vi "getSigProcessing.vi"(0 "Analogue Data (volts)":dbl[][](array[numeric])) -> (1 "Labelled Signals":string[][](array[string]), 2 "Channel Names":string[](array[string]), 3 "Raw Signals":dbl[][](array[numeric]))   [LabVIEW 2013]
uses:
  Globals/measurementGlobal.vi
panel:
  out "Chell Chans.":dbl[](array[numeric])
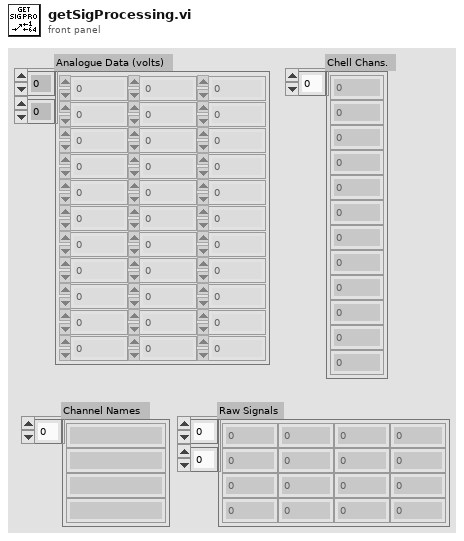
[diagram p1: front panel]
types:
  T1 = typedef "chanType.ctl" = enum16{"Default", "Clock", "Pressure Scanner"}
  T2 = typedef "chanData.ctl" = cluster{"Raw Data":dbl[], "Channel Name":string}
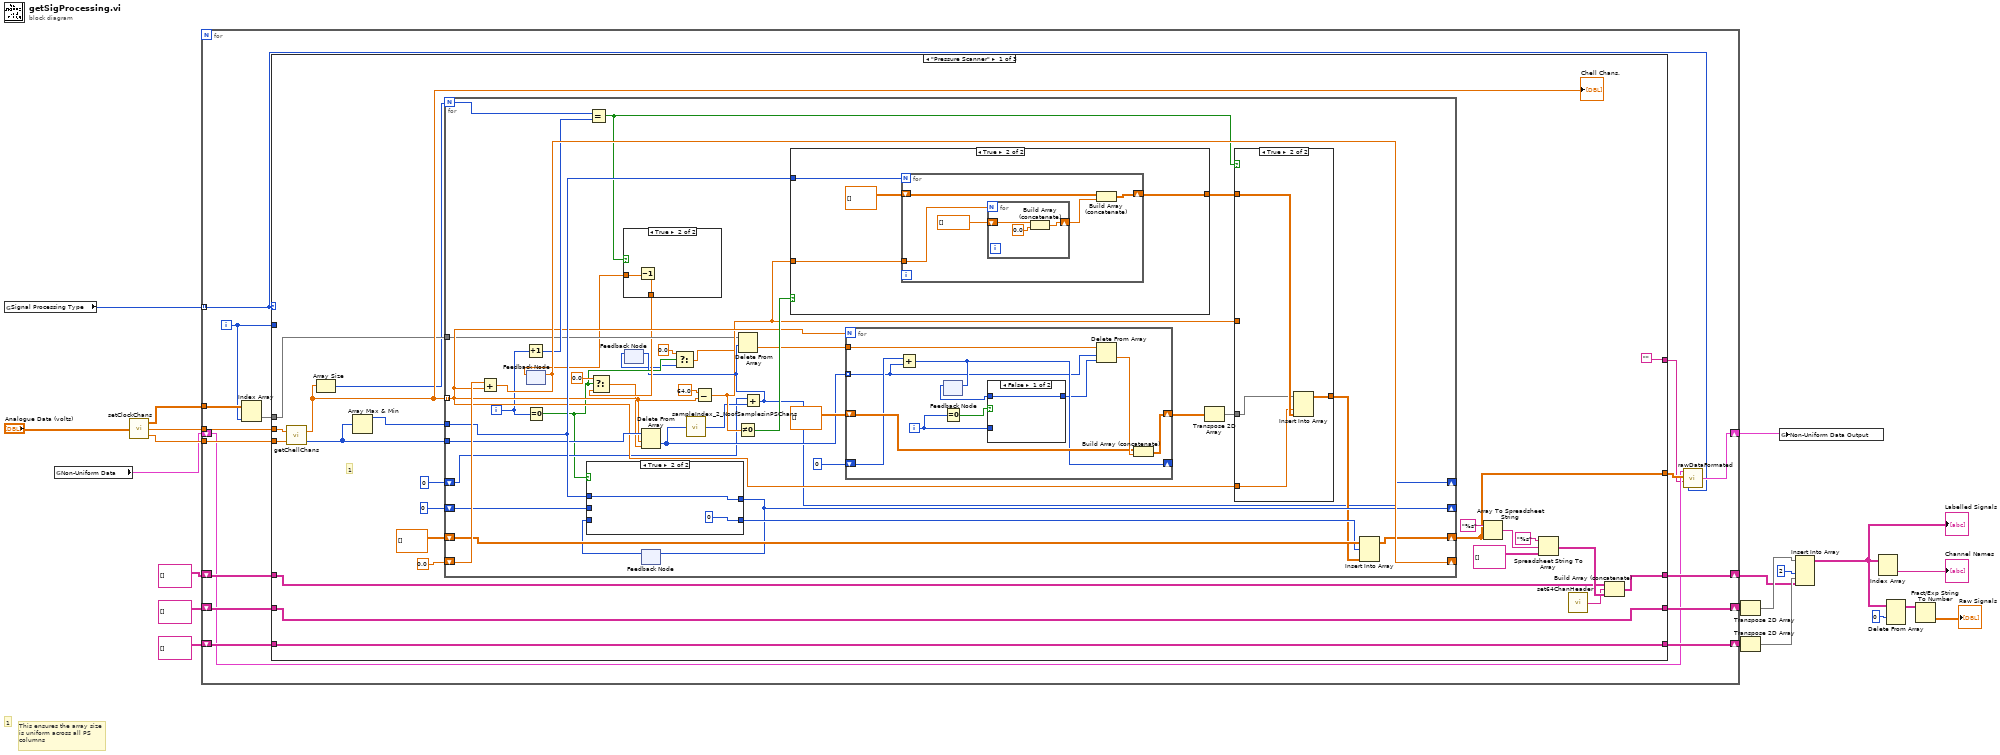
[diagram p0: block diagram]
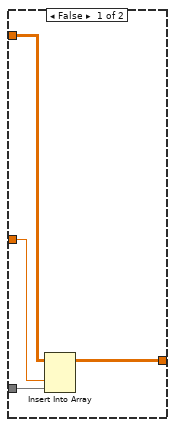
[diagram p3: hidden frame]
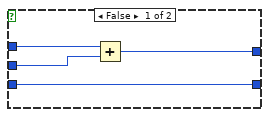
[diagram p4: hidden frame]
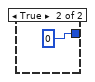
[diagram p5: hidden frame]
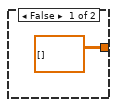
[diagram p6: hidden frame]
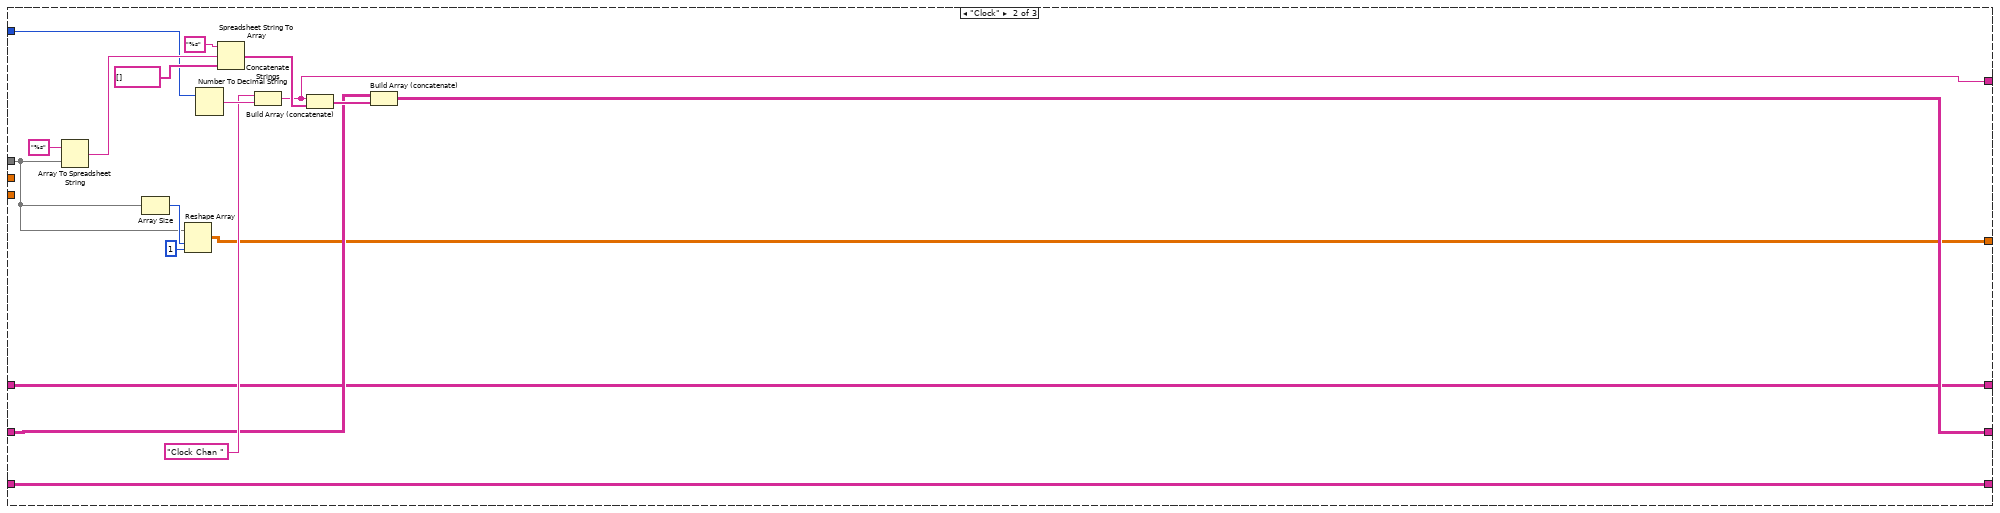
[diagram p7: hidden frame]
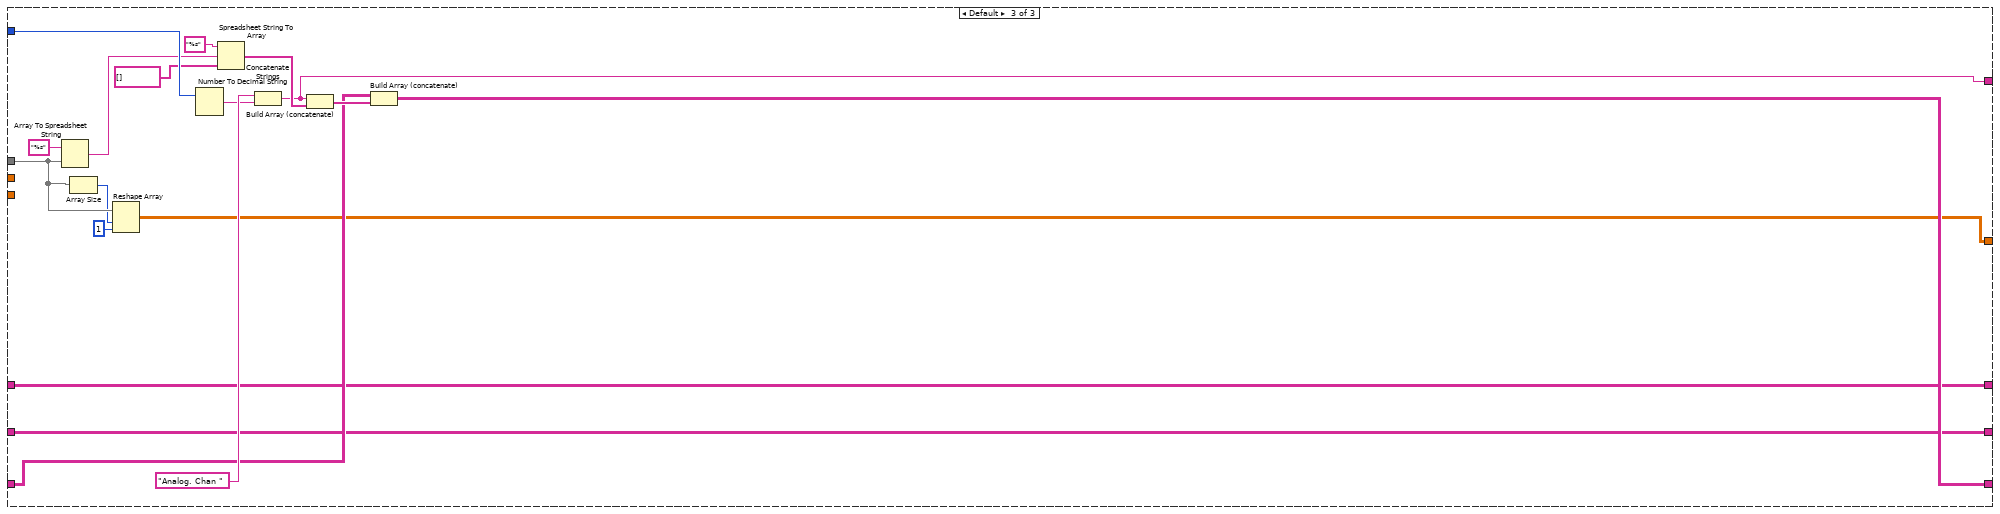
[diagram p8: hidden frame]
diagram:
  # "1"
  # "This ensures the array size\nis uniform across all PS\ncolumns"
  n1 = global read "measurementGlobal.vi" "Signal Processing Type"() -> (w21:T1[])
  n2 = global read "measurementGlobal.vi" "Non-Uniform Data"() -> (w2:T2[])
  n3 = call "setClockChans.vi"("Analogue Data (volts)"="Analogue Data (volts)") -> ("Modified Analogue Data (volts)"=w14:dbl[][], "MSB"=w13:dbl[], "LSB"=w12:dbl[])
  n4 = for {
    tunnel: w21 -> [w22] mode=indexing
    tunnel: w14 -> [w36]
    tunnel: w13 -> [w35]
    tunnel: w12 -> [w34]
    shift-right: [w31] -> w9
    shift-left: string[][] [] -> [w32]
    shift-right: [w29] -> w5
    shift-left: string[][] [] -> [w30]
    shift-right: [w27] -> w3
    shift-left: string[][] [] -> [w28]
    shift-right: [w25] -> w1
    shift-left: w2 -> [w24]
    i -> [w33]
    n5 = Index Array(array=w36, index (col)=w33) -> (element=w37:dbl[])  [unwired: 1 in]
    n6 = case shown="\"Pressure Scanner\"" w22 {
      tunnel: w37 -> [w52 w144 w163]
      tunnel: w35 -> [w60 _ _]
      tunnel: w34 -> [w59 _ _]
      tunnel: w33 -> [_ w152 w176]
      tunnel: w32 -> [w46 w150 w166]
      tunnel: [w46 w149 w166] -> w31
      tunnel: w30 -> [w45 w148 w168]
      tunnel: [w45 w148 w167] -> w29
      tunnel: w28 -> [w44 w147 w165]
      tunnel: [w43 w147 w165] -> w27
      tunnel: [w40 w143 w161] -> w26
      tunnel: ["" w142 w160] -> w23
      frame "Pressure Scanner" {
        # "1"
        n7 = call "getChellChans.vi"("LSB"=w59, "MSB"=w60) -> ("Sample Index"=w58:i32[], "No. Chell Chans."=w55:dbl[])
        "Chell Chans." <- w55
        n8 = Array Size(array=w55) -> (size(s)=w42:i32)
        n9 = Array Max & Min(array=w58) -> (max value=w57:i32)  [unwired: 3 out]
        n10 = for {
          N: w42 -> [w85]
          tunnel: w55 -> [w82] mode=indexing
          tunnel: w52 -> [w77]
          tunnel: w58 -> [w87]
          tunnel: w57 -> [w92]
          shift-right: [w94] -> _
          shift-left: 0.0 -> [w95]
          shift-right: [w61] -> w40
          shift-left: dbl[][] [] ("array") -> [w93]
          shift-right: [w89] -> _
          shift-left: 0 -> [w90]
          shift-right: [w64] -> _
          shift-left: 0 -> [w67]
          i -> [w79]
          n11 = Add(x=w95, y=w82) -> (x+y=w94:dbl)
          n12 = Increment(x=w79) -> (x+1=w84:i32)
          n13 = feedback #1() -> (w72:dbl)  [unwired: 1 in]
          n14 = feedback-in #1(w94) -> ()
          n15 = Equal To 0?(x=w79) -> (x = 0?=w66:bool)
          n16 = Equal?(x=w85, y=w84) -> (x = y?=w73:bool)
          n17 = case shown="True" w73 {
            tunnel: w72 -> [w99 w101]
            tunnel: [w99 w100] -> w70
            frame False {
            }
            frame True {
              n18 = Decrement(x=w101) -> (x-1=w100:dbl)
            }
          }
          n19 = Select(t=0.0, s=w66, f=w70) -> (s? t:f=w69:dbl)
          n20 = feedback #2() -> (w63:i32)  [unwired: 1 in]
          n21 = Delete From Array(array=w87, length=w82, index=w69) -> (deleted portion=w74:i32[])  [unwired: 1 out]
          n22 = feedback #3() -> (w88:i32)  [unwired: 1 in]
          n23 = case shown="True" w66 {
            tunnel: w92 -> [w112 w115]
            tunnel: [w110 0] -> w91
            tunnel: w90 -> [w113 _]
            tunnel: [w111 w115] -> w89
            tunnel: w88 -> [w110 _]
            frame False {
              n24 = Add(x=w112, y=w113) -> (x+y=w111:i32)
            }
            frame True {
            }
          }
          n25 = feedback-in #3(w89) -> ()
          n26 = Select(t=0.0, s=w66, f=w63) -> (s? t:f=w62:dbl)
          n27 = call "sampleIndex_2_NoofSamplesinPSChans.vi"("Sample Index"=w74) -> ("No of Samples in PS Chans"=w68:i32)
          n28 = Subtract(x=64.0 ("y"), y=w82) -> (x-y=w81:dbl)
          n29 = Not Equal To 0?(x=w81) -> (x != 0?=w86:bool)
          n30 = Add(x=w67, y=w68) -> (x+y=w64:i32)
          n31 = feedback-in #2(w64) -> ()
          n32 = Delete From Array(array=w77, length=w64, index=w62) -> (deleted portion=w76:dbl[])  [unwired: 1 out]
          n33 = case shown="True" w86 {
            tunnel: w81 -> [_ w130]
            tunnel: [dbl[][] [] w133] -> w83
            tunnel: w92 -> [_ w132]
            frame False {
            }
            frame True {
              n34 = for {
                N: w132 -> [_]
                shift-right: [w135] -> w133
                shift-left: dbl[][] [] -> [w136]
                tunnel: w130 -> [w134]
                n35 = for {
                  N: w134 -> [_]
                  shift-right: [w140] -> w137
                  shift-left: dbl[] [] -> [w141]
                  n36 = Build Array (concatenate)(w141, 0.0) -> (w140:dbl[])
                }
                n37 = Build Array (concatenate)(w136, w137) -> (w135:dbl[][])
              }
            }
          }
          n38 = for {
            N: w82 -> [_]
            tunnel: w74 -> [w119] mode=indexing
            tunnel: w76 -> [w126]
            shift-right: [w124] -> w78
            shift-left: dbl[][] [] ("element") -> [w123]
            shift-right: [w121] -> _
            shift-left: 0 -> [w122]
            i -> [w118]
            n39 = Add(x=w122, y=w119) -> (x+y=w121:i32)
            n40 = feedback-in #4(w121) -> ()
            n41 = feedback #4() -> (w120:i32)  [unwired: 1 in]
            n42 = Equal To 0?(x=w118) -> (x = 0?=w117:bool)
            n43 = case shown="False" w117 {
              tunnel: [w127 0] -> w116
              tunnel: w118 -> [_ _]
              tunnel: w120 -> [w127 _]
              frame False {
              }
              frame True {
              }
            }
            n44 = Delete From Array(array=w126, length=w119, index=w116) -> (deleted portion=w125:dbl[])  [unwired: 1 out]
            n45 = Build Array (concatenate)(w123, w125) -> (w124:dbl[][])
          }
          n46 = Transpose 2D Array(2D array=w78) -> (transposed array=w75:dbl[][])
          n47 = case shown="True" w73 {
            tunnel: w83 -> [w105 w109]
            tunnel: w75 -> [w104 w108]
            tunnel: w82 -> [_ w106]
            tunnel: w81 -> [w103 _]
            tunnel: [w102 w107] -> w80
            frame False {
              n48 = Insert Into Array(array=w105, index (col)=w103, new element=w104) -> (w102:dbl[][])  [unwired: 1 in]
            }
            frame True {
              n49 = Insert Into Array(array=w108, index (col)=w106, new element=w109) -> (w107:dbl[][])  [unwired: 1 in]
            }
          }
          n50 = Insert Into Array(array=w93, index (row)=w91, new element=w80) -> (w61:dbl[][])  [unwired: 1 in]
        }
        n51 = Array To Spreadsheet String(array=w40, 3:"%s" ("format string")) -> (spreadsheet string=w50:string)  [unwired: 1 in]
        n52 = Spreadsheet String To Array(format string="%s", spreadsheet string=w50, array type (2D Dbl)=string[][] []) -> (array=w47:string[][])  [unwired: 1 in]
        n53 = call "set64ChanHeader.vi"() -> ("64 Chan Header"=w39:string[])
        n54 = Build Array (concatenate)(w44, w39, w47) -> (w43:string[][])
      }
      frame "Clock" {
        n55 = Array To Spreadsheet String(array=w144, 3:"%s" ("format string")) -> (spreadsheet string=w156:string)  [unwired: 1 in]
        n56 = Array Size(array=w144) -> (size(s)=w145:i32)
        n57 = Reshape Array(w144, w145, 1 ("dimension size")) -> (w143:dbl[][])
        n58 = Number To Decimal String(number=w152) -> (decimal integer string=w154:string)  [unwired: 1 in]
        n59 = Spreadsheet String To Array(format string="%s", spreadsheet string=w156, array type (2D Dbl)=string[] []) -> (array=w159:string[])  [unwired: 1 in]
        n60 = Concatenate Strings("Clock Chan " ("string"), w154) -> (w142:string)
        n61 = Build Array (concatenate)(w142, w159) -> (w151:string[])
        n62 = Build Array (concatenate)(w150, w151) -> (w149:string[][])
      }
      frame Default {
        n63 = Array To Spreadsheet String(array=w163, 3:"%s" ("format string")) -> (spreadsheet string=w173:string)  [unwired: 1 in]
        n64 = Array Size(array=w163) -> (size(s)=w162:i32)
        n65 = Reshape Array(w163, w162, 1 ("dimension size")) -> (w161:dbl[][])
        n66 = Number To Decimal String(number=w176) -> (decimal integer string=w175:string)  [unwired: 1 in]
        n67 = Spreadsheet String To Array(format string="%s", spreadsheet string=w173, array type (2D Dbl)=string[] []) -> (array=w170:string[])  [unwired: 1 in]
        n68 = Concatenate Strings("Analog. Chan " ("string"), w175) -> (w160:string)
        n69 = Build Array (concatenate)(w160, w170) -> (w169:string[])
        n70 = Build Array (concatenate)(w168, w169) -> (w167:string[][])
      }
    }
    n71 = call "rawDataFormated.vi"("Channel Type"=w22, "Channel Name"=w23, "2D Data"=w26, "Non-Uniform Data"=w24) -> ("Non-Uniform Data Output"=w25:T2[])
  }
  n72 = Transpose 2D Array(2D array=w9) -> (transposed array=w7:string[][])
  n73 = Transpose 2D Array(2D array=w5) -> (transposed array=w4:string[][])
  n74 = global write "measurementGlobal.vi" "Non-Uniform Data Output"(w1) -> ()
  n75 = Insert Into Array(array=w7, index (col)=2 ("disabled index (col)"), new element #1=w4, new element #2=w3) -> (w16:string[][])  [unwired: 1 in]
  "Labelled Signals" <- w16
  n76 = Index Array(array=w16) -> (element=→"Channel Names":string[])  [unwired: 2 in]
  n77 = Delete From Array(array=w16, index (row)=0) -> (array with subset deleted=w18:string[][])  [unwired: 2 in, 1 out]
  n78 = Fract/Exp String To Number(string=w18) -> (number=→"Raw Signals":dbl[][])  [unwired: 3 in, 1 out]
